vi "Knobphase.vi"(0 "Freqin":dbl=1000.0 format="%_7g", 2 "Knob":i8(knob)=1 scale=1.0..20.0, 3 "Step Size":dbl, 4 "Reset":bool, 5 "pup":bool, 6 "pdn":bool) -> (8 "Freqout":dbl format="%_7g", 10 "Phase Pr Out":dbl)   [LabVIEW 2012]
panel:
  out "x-y":dbl
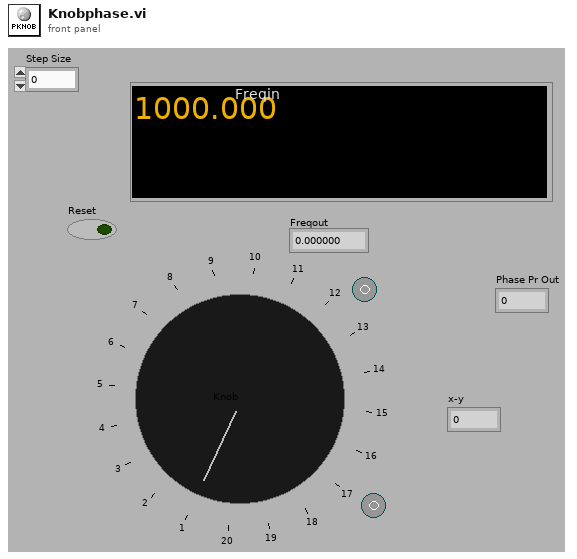
[diagram p1: front panel]
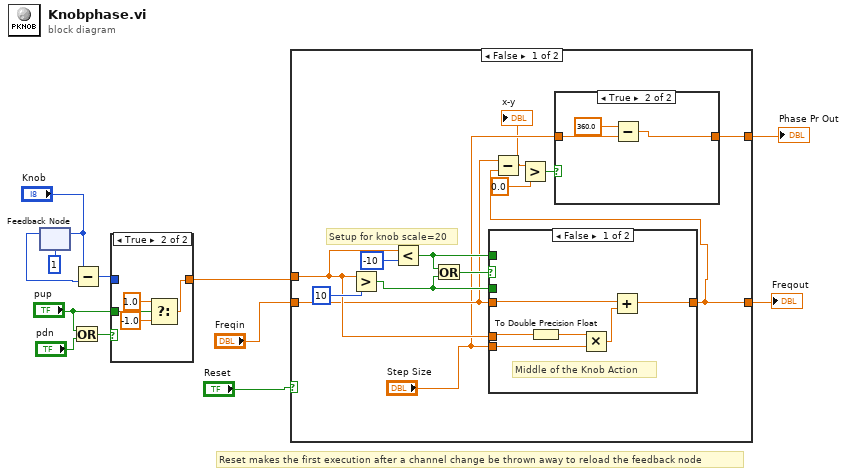
[diagram p0: block diagram]
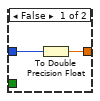
[diagram p2: hidden frame]
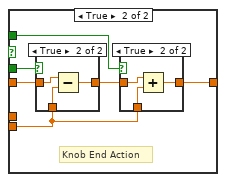
[diagram p4: hidden frame]
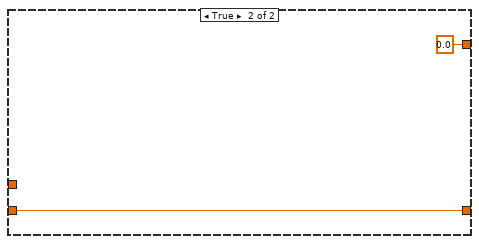
[diagram p7: hidden frame]
diagram:
  # "Reset makes the first execution after a channel change be thrown away to reload the feedback node"
  n1 = feedback-in #1("Knob") -> ()
  n2 = feedback #1(i8 1 ("Knob")) -> (w11:i8)
  n3 = Or(x="pup", y="pdn") -> (x .or. y?=w5:bool)
  n4 = Subtract(x="Knob", y=w11) -> (x-y=w4:i8)
  n5 = case shown="True" w5 {
    tunnel: w4 -> [w13 _]
    tunnel: [w14 w17] -> w3
    tunnel: "pup" -> [_ w18]
    frame False {
      n6 = To Double Precision Float(number=w13) -> (double precision float=w14:dbl)
    }
    frame True {
      n7 = Select(t=1.0, s=w18, f=-1.0) -> (s? t:f=w17:dbl)
    }
  }
  n8 = case shown="False" "Reset" {
    tunnel: w3 -> [w26 _]
    tunnel: "Freqin" -> [w25 w57]
    tunnel: [w19 w57] -> w8
    tunnel: [w22 0.0 ("Step Size")] -> w6
    frame False {
      # "Setup for knob scale=20"
      n9 = Greater?(x=w26, y=10) -> (0:w28:bool)
      n10 = Less?(x=w26, y=-10) -> (x < y?=w27:bool)
      n11 = Or(x=w27, y=w28) -> (x .or. y?=w29:bool)
      n12 = case shown="False" w29 {
        tunnel: w28 -> [_ w47]
        tunnel: w25 -> [w40 w46]
        tunnel: w27 -> [_ w44]
        tunnel: [w41 w43] -> w19
        tunnel: "Step Size" -> [w36 w42]
        tunnel: w26 -> [w37 _]
        frame False {
          # "Middle of the Knob Action"
          n13 = To Double Precision Float(number=w37) -> (double precision float=w38:dbl)
          n14 = Multiply(x=w38, y=w36) -> (x*y=w39:dbl)
          n15 = Add(x=w40, y=w39) -> (x+y=w41:dbl)
        }
        frame True {
          # "Knob End Action"
          n16 = case shown="True" w47 {
            tunnel: w46 -> [w52 w54]
            tunnel: [w52 w55] -> w45
            tunnel: w42 -> [_ w53]
            frame False {
            }
            frame True {
              n17 = Subtract(x=w54, y=w53) -> (x-y=w55:dbl)
            }
          }
          n18 = case shown="True" w44 {
            tunnel: w45 -> [w48 w50]
            tunnel: [w48 w51] -> w43
            tunnel: w42 -> [_ w49]
            frame False {
            }
            frame True {
              n19 = Add(x=w50, y=w49) -> (x+y=w51:dbl)
            }
          }
        }
      }
      n20 = Subtract(x=w25, y=w19) -> (x-y=w21:dbl)
      "x-y" <- w21
      n21 = Greater?(x=w21, y=0.0) -> (0:w24:bool)
      n22 = case shown="True" w24 {
        tunnel: "Step Size" -> [w32 w35]
        tunnel: [w32 w33] -> w22
        frame False {
        }
        frame True {
          n23 = Subtract(x=360.0, y=w35) -> (x-y=w33:dbl)
        }
      }
    }
    frame True {
    }
  }
  "Freqout" <- w8
  "Phase Pr Out" <- w6
